vi "myRIO_BRig_Host_formatData_test1.vi"(7 "input_filePath":string, 8 "input_error":errorcluster, 9 "input_data":u16[][](array[numeric]), 10 "input_headers":string[](array[string]), 11 "input_hdl_Workbooks":refnum<k7>) -> (0 "output_error":errorcluster, 3 "output_hdl_Worksbooks":refnum<k7>)   [LabVIEW 2014]
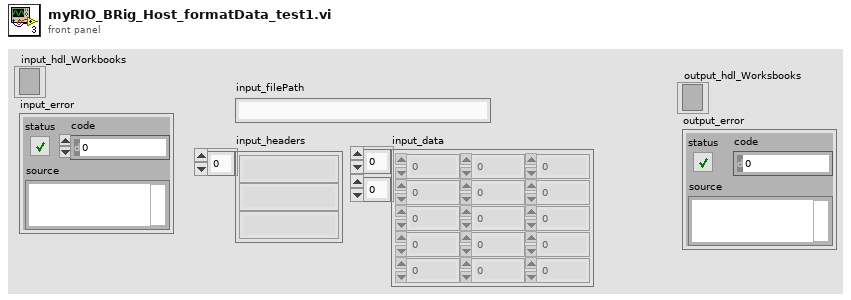
[diagram p1: front panel]
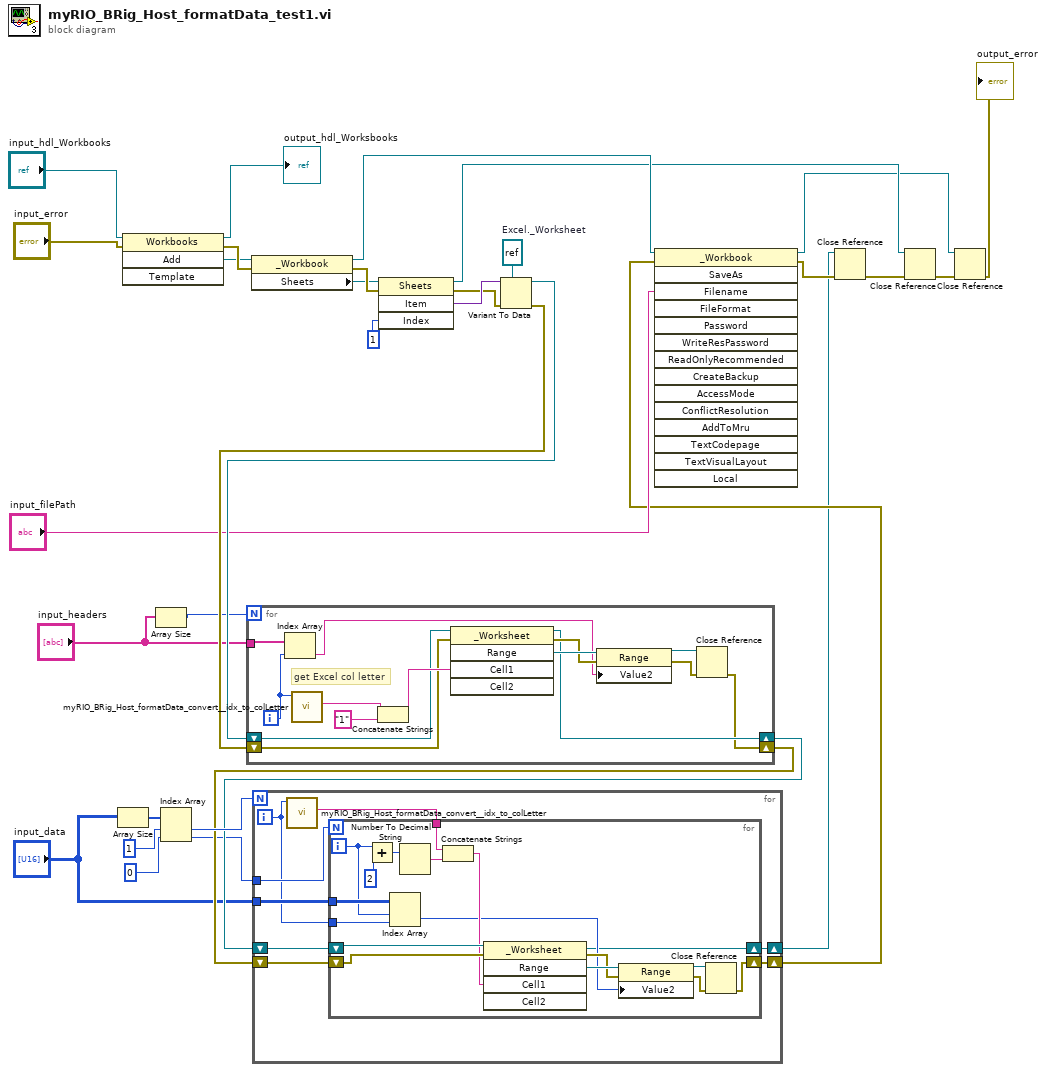
[diagram p0: block diagram]
diagram:
  w28 = refnum<k7> refnum  # Excel._Worksheet
  n1 = Array Size(array="input_data") -> (size(s)=w14:i32[])
  n2 = invoke class="Workbooks" method="Add"(reference="input_hdl_Workbooks", error in="input_error") -> (reference out=→"output_hdl_Worksbooks":refnum<k7>, error out=w32:errorcluster, "Add"=w30:refnum<k7>)  [unwired: 2 in, 1 out]
  n3 = Array Size(array="input_headers") -> (size(s)=w15:i32)
  n4 = Index Array(array=w14, index #1=1 ("index"), index #2=0 ("index")) -> (element #1=w11:i32, element #2=w8:i32)
  n5 = property class="_Workbook"(reference=w30, error in=w32) -> (reference out=w25:refnum<k7>, error out=w33:errorcluster, "Sheets"=w29:refnum<k7>)
  n6 = invoke class="Sheets" method="Item"(reference=w29, error in=w33, "Index"=1) -> (reference out=w24:refnum<k7>, error out=w26:errorcluster, "Item"=w27:variant)  [unwired: 1 in, 1 out]
  n7 = Variant To Data(error in=w26, type=w28, Variant=w27) -> (data=w18:refnum<k7>, error out=w19:errorcluster)
  n8 = for {
    N: w15 -> [_]
    tunnel: "input_headers" -> [w47]
    shift-right: [w37] -> w9
    shift-left: w18 -> [w39]
    shift-right: [w34] -> w10
    shift-left: w19 -> [w38]
    i -> [w46]
    # "get Excel col letter"
    n9 = Index Array(array=w47, index=w46) -> (element=w40:string)
    n10 = call "myRIO_BRig_Host_formatData_convert__idx_to_colLetter.vi"("input_idx"=w46) -> ("output_colLetter"=w44:string)  [unwired: 10 in]
    n11 = Concatenate Strings(w44, "1" ("string")) -> (w43:string)
    n12 = invoke class="_Worksheet" method="Range"(reference=w39, error in=w38, "Cell1"=w43) -> (reference out=w37:refnum<k7>, error out=w41:errorcluster, "Range"=w42:refnum<k7>)  [unwired: 2 in, 2 out]
    n13 = property class="Range"(reference=w42, error in=w41, "Value2"=w40) -> (reference out=w36:refnum<k7>, error out=w35:errorcluster)
    n14 = Close Reference(reference=w36, error in (no error)=w35) -> (error out=w34:errorcluster)
  }
  n15 = for {
    N: w11 -> [_]
    shift-right: [w49] -> w6
    shift-left: w10 -> [w55]
    shift-right: [w48] -> w5
    shift-left: w9 -> [w54]
    tunnel: w8 -> [w53]
    tunnel: "input_data" -> [w51]
    i -> [w50]
    n16 = call "myRIO_BRig_Host_formatData_convert__idx_to_colLetter.vi"("input_idx"=w50) -> ("output_colLetter"=w52:string)  [unwired: 10 in]
    n17 = for {
      N: w53 -> [_]
      shift-right: [w57] -> w49
      shift-left: w55 -> [w64]
      shift-right: [w56] -> w48
      shift-left: w54 -> [w65]
      tunnel: w52 -> [w69]
      tunnel: w51 -> [w68]
      tunnel: w50 -> [w66]
      i -> [w67]
      n18 = Add(x=w67, y=2 ("string")) -> (x+y=w71:i32)
      n19 = Index Array(array=w68, index (row)=w67, index (col)=w66) -> (element=w60:u16)
      n20 = Number To Decimal String(number=w71) -> (decimal integer string=w70:string)  [unwired: 1 in]
      n21 = Concatenate Strings(w69, w70) -> (w63:string)
      n22 = invoke class="_Worksheet" method="Range"(reference=w65, error in=w64, "Cell1"=w63) -> (reference out=w56:refnum<k7>, error out=w61:errorcluster, "Range"=w62:refnum<k7>)  [unwired: 2 in, 2 out]
      n23 = property class="Range"(reference=w62, error in=w61, "Value2"=w60) -> (reference out=w59:refnum<k7>, error out=w58:errorcluster)
      n24 = Close Reference(reference=w59, error in (no error)=w58) -> (error out=w57:errorcluster)
    }
  }
  n25 = invoke class="_Workbook" method="SaveAs"(reference=w25, error in=w6, "Filename"="input_filePath") -> (reference out=w20:refnum<k7>, error out=w22:errorcluster)  [unwired: 12 in, 13 out]
  n26 = Close Reference(reference=w5, error in (no error)=w22) -> (error out=w23:errorcluster)
  n27 = Close Reference(reference=w24, error in (no error)=w23) -> (error out=w21:errorcluster)
  n28 = Close Reference(reference=w20, error in (no error)=w21) -> (error out=→"output_error":errorcluster)
